vi "TestExec.Deploy Sequence Folders and Files.vi"(9 "Destination Folder":path=path "C:/MTE/Laser Module Test/Sequences", 11 "Source Folder":path) -> ()   [LabVIEW 2019]
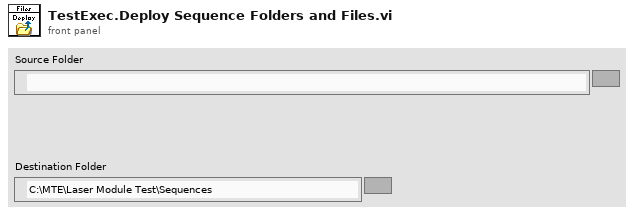
[diagram p1: front panel]
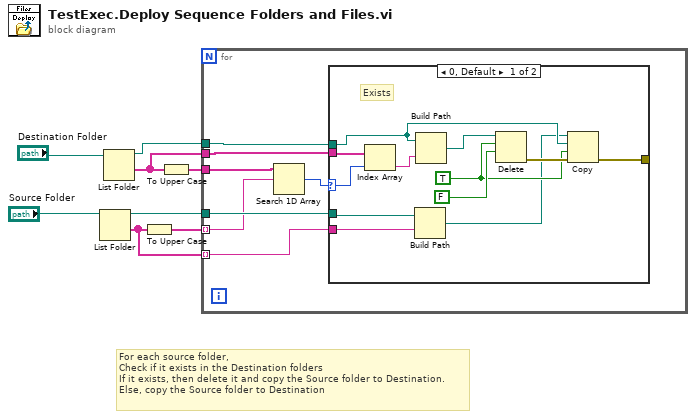
[diagram p0: block diagram]
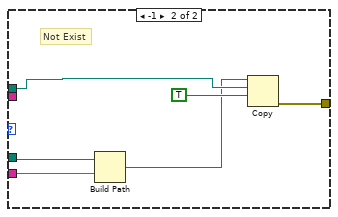
[diagram p2: hidden frame]
diagram:
  # "For each source folder, \nCheck if it exists in the Destination folders\nIf it exists, then delete it and copy the Source folder to Destination.\nElse, copy the Source folder to Destination"
  n1 = List Folder(path="Source Folder") -> (path out=w7:path, folder names=w1:string[])  [unwired: 3 in, 2 out]
  n2 = List Folder(path="Destination Folder") -> (path out=w5:path, folder names=w2:string[])  [unwired: 3 in, 2 out]
  n3 = To Upper Case(1:w1) -> (0:w4:string[])
  n4 = To Upper Case(1:w2) -> (0:w3:string[])
  n5 = for {
    tunnel: w7 -> [w12]
    tunnel: w5 -> [w13]
    tunnel: w4 -> [w11] mode=indexing
    tunnel: w3 -> [w14]
    tunnel: w2 -> [w10]
    tunnel: w1 -> [w9] mode=indexing
    n6 = Search 1D Array(1D array=w14, element=w11) -> (index of element=w15:i32)  [unwired: 1 in]
    n7 = case shown="0, Default" w15 {
      selector: w15 -> [w26 _]
      tunnel: w10 -> [w27 _]
      tunnel: w13 -> [w17 w29]
      tunnel: w12 -> [w19 w31]
      tunnel: w9 -> [w18 w30]
      tunnel: [w20 w32] -> _
      frame 0, Default {
        w21 = TRUE ("entire hierarchy (F)")
        # "Exists"
        n8 = Index Array(array=w27, index=w26) -> (element=w25:string)
        n9 = Build Path(base path=w19, name or relative path=w18) -> (appended path=w16:path)
        n10 = Build Path(base path=w17, name or relative path=w25) -> (appended path=w24:path)
        n11 = Delete(path (use dialog)=w24, entire hierarchy (F)=w21, confirm (F)=FALSE ("entire hierarchy (F)")) -> (error out=w22:errorcluster)  [unwired: 2 in, 2 out]
        n12 = Copy(8:w22, 9:w21, 10:w17, 11:w16) -> (0:w20:errorcluster)  [unwired: 1 in, 2 out]
      }
      frame -1 {
        # "Not Exist"
        n13 = Build Path(base path=w31, name or relative path=w30) -> (appended path=w28:path)
        n14 = Copy(9:TRUE ("entire hierarchy (F)"), 10:w29, 11:w28) -> (0:w32:errorcluster)  [unwired: 2 in, 2 out]
      }
    }
  }
